vi "Test_01.vi"() -> ()   [LabVIEW 2015]
panel:
  in  "Stop Application":bool
  in  "Stop Button":bool
  out "Chart":dbl(graph)
  out "Graph":dbl[](graph)
  in  "Continious":bool
  in  "Enum":enum16{"Sine", "Sawtooth", "Square"}(ring)
  in  "Period multiplier":dbl=1.0
  in  "Amplitude":dbl=1.0
  in  "Periods to generate":dbl=1.0
  in  "Generate":bool
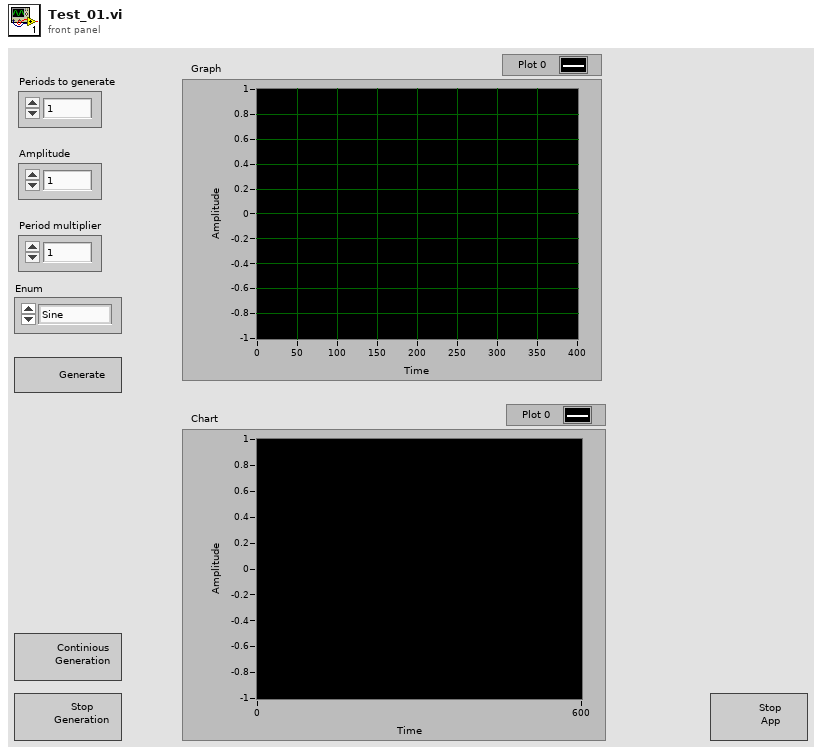
[diagram p1: front panel]
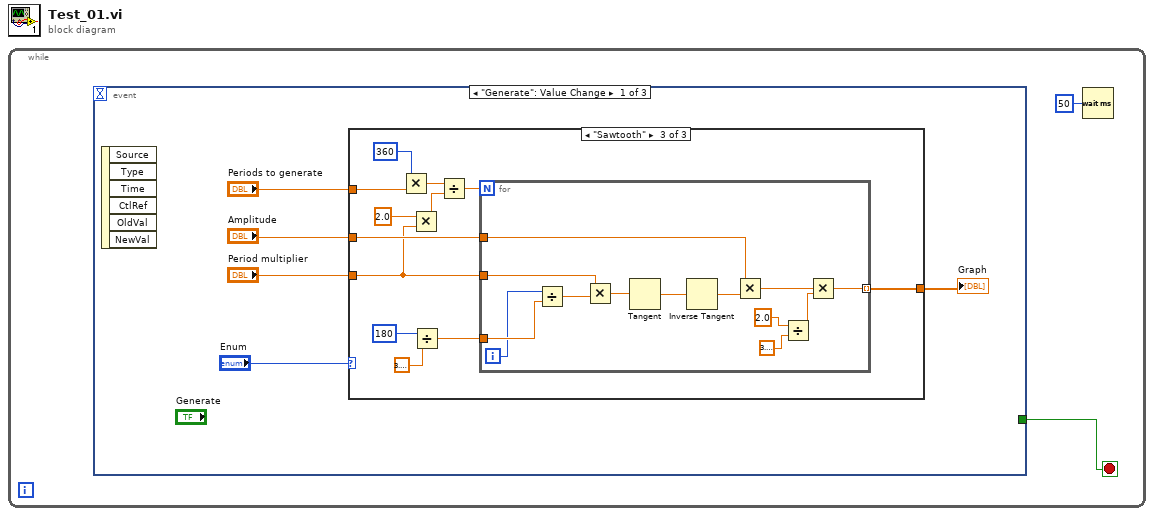
[diagram p0: block diagram]
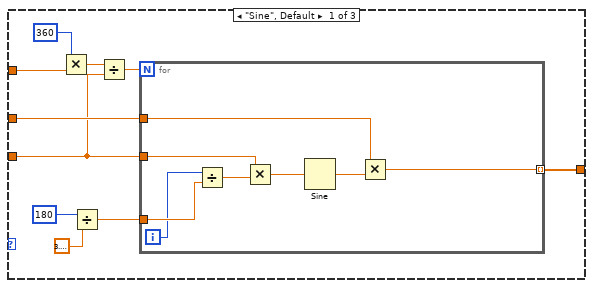
[diagram p2: hidden frame]
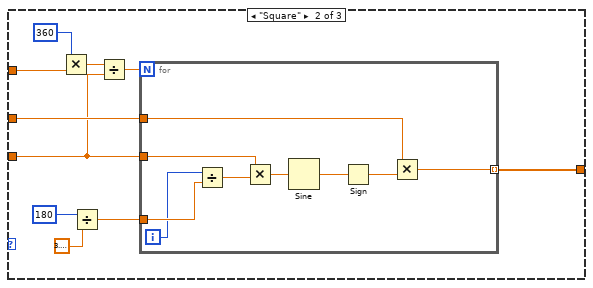
[diagram p3: hidden frame]
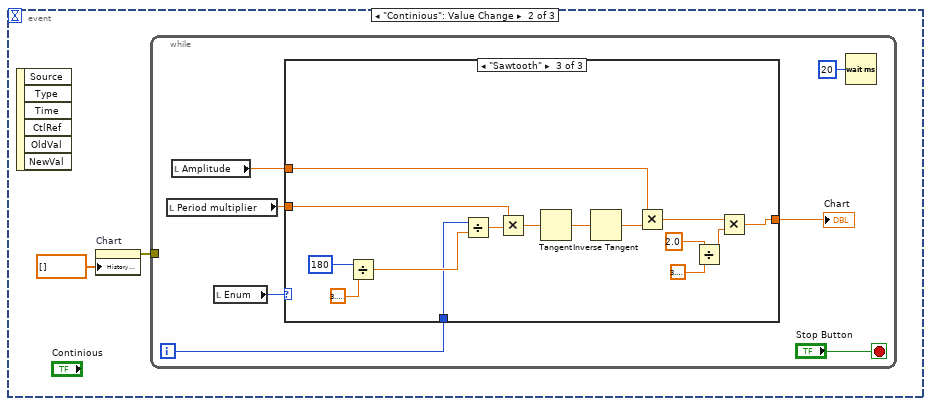
[diagram p4: hidden frame]
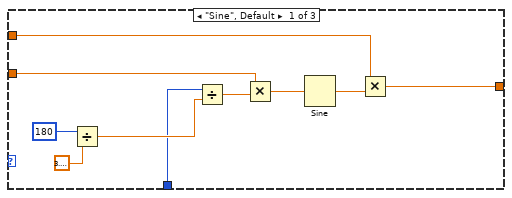
[diagram p5: hidden frame]
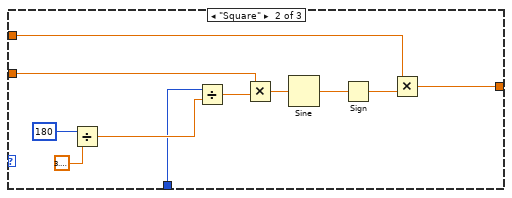
[diagram p6: hidden frame]
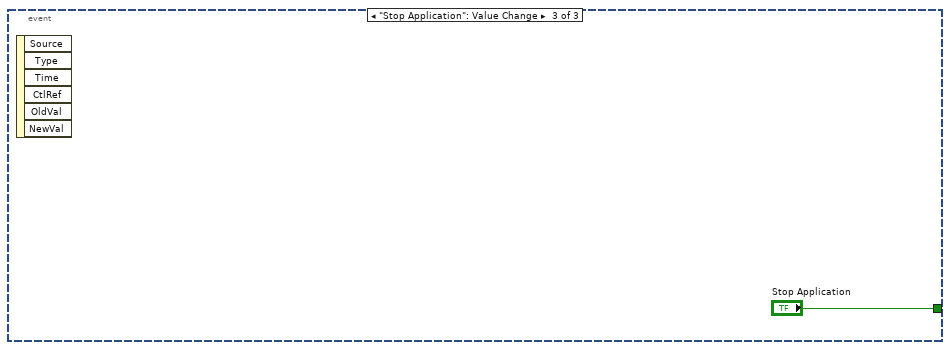
[diagram p7: hidden frame]
diagram:
  n1 = while {
    stop <- w1 stop-if-true
    n2 = event shown="[0] \"Generate\": Value Change" {
      selector: _ -> [_ _ _]
      dyn-events: _ -> [_ _ _]
      timeout: _ -> [_ _ _]
      tunnel: [_ _ "Stop Application"] -> w1
      event "Generate": Value Change {
        n3 = event-data() -> ()  [unwired: 1 in, 6 out]
        n4 = case shown="\"Sawtooth\"" "Enum" {
          tunnel: "Periods to generate" -> [w13 w31 w52]
          tunnel: "Period multiplier" -> [w10 w28 w48]
          tunnel: "Amplitude" -> [w12 w30 w51]
          tunnel: [w8 w26 w45] -> w3
          frame "Sine", Default {
            n5 = Multiply(x=360, y=w13) -> (x*y=w11:dbl)
            n6 = Divide(x=180, y=3.141592653589793) -> (x/y=w14:dbl)
            n7 = Divide(x=w11, y=w10) -> (x/y=w9:dbl)
            n8 = for {
              N: w9 -> [_]
              tunnel: w14 -> [w25]
              tunnel: w10 -> [w19]
              tunnel: w12 -> [w23]
              tunnel: [w18] -> w8 mode=indexing
              i -> [w22]
              n9 = Divide(x=w22, y=w25) -> (x/y=w21:dbl)
              n10 = Multiply(x=w19, y=w21) -> (x*y=w20:dbl)
              n11 = Sine(x=w20) -> (sin(x)=w24:dbl)
              n12 = Multiply(x=w23, y=w24) -> (x*y=w18:dbl)
            }
          }
          frame "Square" {
            n13 = Multiply(x=360, y=w31) -> (x*y=w29:dbl)
            n14 = Divide(x=180, y=3.141592653589793) -> (x/y=w32:dbl)
            n15 = Divide(x=w29, y=w28) -> (x/y=w27:dbl)
            n16 = for {
              N: w27 -> [_]
              tunnel: w32 -> [w44]
              tunnel: w28 -> [w39]
              tunnel: w30 -> [w43]
              tunnel: [w36] -> w26 mode=indexing
              i -> [w42]
              n17 = Divide(x=w42, y=w44) -> (x/y=w41:dbl)
              n18 = Multiply(x=w39, y=w41) -> (x*y=w40:dbl)
              n19 = Sine(x=w40) -> (sin(x)=w38:dbl)
              n20 = Sign(1:w38) -> (0:w37:dbl)
              n21 = Multiply(x=w43, y=w37) -> (x*y=w36:dbl)
            }
          }
          frame "Sawtooth" {
            n22 = Multiply(x=360, y=w52) -> (x*y=w50:dbl)
            n23 = Multiply(x=2.0, y=w48) -> (x*y=w46:dbl)
            n24 = Divide(x=180, y=3.141592653589793) -> (x/y=w53:dbl)
            n25 = Divide(x=w50, y=w46) -> (x/y=w49:dbl)
            n26 = for {
              N: w49 -> [_]
              tunnel: w53 -> [w69]
              tunnel: w48 -> [w65]
              tunnel: w51 -> [w68]
              tunnel: [w57] -> w45 mode=indexing
              i -> [w67]
              n27 = Divide(x=w67, y=w69) -> (x/y=w66:dbl)
              n28 = Multiply(x=w65, y=w66) -> (x*y=w64:dbl)
              n29 = Tangent(1:w64) -> (0:w63:dbl)
              n30 = Inverse Tangent(1:w63) -> (0:w62:dbl)
              n31 = Multiply(x=w68, y=w62) -> (x*y=w61:dbl)
              n32 = Divide(x=2.0, y=3.141592653589793) -> (x/y=w58:dbl)
              n33 = Multiply(x=w61, y=w58) -> (x*y=w57:dbl)
            }
          }
        }
        "Graph" <- w3
      }
      event "Continious": Value Change {
        n34 = event-data() -> ()  [unwired: 1 in, 6 out]
        n35 = property on="Chart" class="WFChart (strict)"("History Data"=dbl[] []) -> (error out=w70:errorcluster)  [unwired: 2 in, 1 out]
        n36 = while {
          tunnel: w70 -> [_]
          i -> [w74]
          stop <- "Stop Button" stop-if-true
          n37 = local read "Period multiplier"() -> (w77:dbl)
          n38 = local read "Amplitude"() -> (w76:dbl)
          n39 = local read "Enum"() -> (w78:enum16{"Sine", "Sawtooth", "Square"})
          n40 = case shown="\"Sawtooth\"" w78 {
            tunnel: w77 -> [w84 w95 w110]
            tunnel: w76 -> [w85 w96 w111]
            tunnel: w74 -> [w80 w90 w105]
            tunnel: [w79 w89 w100] -> w73
            frame "Sine", Default {
              n41 = Divide(x=180, y=3.141592653589793) -> (x/y=w86:dbl)
              n42 = Divide(x=w80, y=w86) -> (x/y=w82:dbl)
              n43 = Multiply(x=w84, y=w82) -> (x*y=w81:dbl)
              n44 = Sine(x=w81) -> (sin(x)=w83:dbl)
              n45 = Multiply(x=w85, y=w83) -> (x*y=w79:dbl)
            }
            frame "Square" {
              n46 = Divide(x=180, y=3.141592653589793) -> (x/y=w97:dbl)
              n47 = Divide(x=w90, y=w97) -> (x/y=w94:dbl)
              n48 = Multiply(x=w95, y=w94) -> (x*y=w93:dbl)
              n49 = Sine(x=w93) -> (sin(x)=w92:dbl)
              n50 = Sign(1:w92) -> (0:w91:dbl)
              n51 = Multiply(x=w96, y=w91) -> (x*y=w89:dbl)
            }
            frame "Sawtooth" {
              n52 = Divide(x=180, y=3.141592653589793) -> (x/y=w112:dbl)
              n53 = Divide(x=w105, y=w112) -> (x/y=w109:dbl)
              n54 = Multiply(x=w110, y=w109) -> (x*y=w108:dbl)
              n55 = Tangent(1:w108) -> (0:w107:dbl)
              n56 = Inverse Tangent(1:w107) -> (0:w106:dbl)
              n57 = Multiply(x=w111, y=w106) -> (x*y=w104:dbl)
              n58 = Divide(x=2.0, y=3.141592653589793) -> (x/y=w101:dbl)
              n59 = Multiply(x=w104, y=w101) -> (x*y=w100:dbl)
            }
          }
          "Chart" <- w73
          n60 = Wait (ms)(milliseconds to wait=u32 20) -> ()  [unwired: 1 out]
        }
      }
      event "Stop Application": Value Change {
        n61 = event-data() -> ()  [unwired: 1 in, 6 out]
      }
    }
    n62 = Wait (ms)(milliseconds to wait=u32 50) -> ()  [unwired: 1 out]
  }
